vi "Receive DS Packet.vi"(0 "Recv Socket":refnum<k16>, 5 "Log User Data":bool) -> (2 "New Dashboard Data":bool, 3 "Battery":sgl, 4 "Error Strings":string, 6 "Driver Station":T1, 8 "Robot IP Address":string="10.0.0.2", 10 "Status":T3, 12 "Camera IP Address":string="10.0.0.2", 13 "Low Priority User Data":string, 14 "High Priority User Data":string, 15 "Error":T2)   [LabVIEW 2014]
uses:
  DStoPCPacketTypeDef.ctl
panel:
  out "CRC":string
  out "Team ID":u16
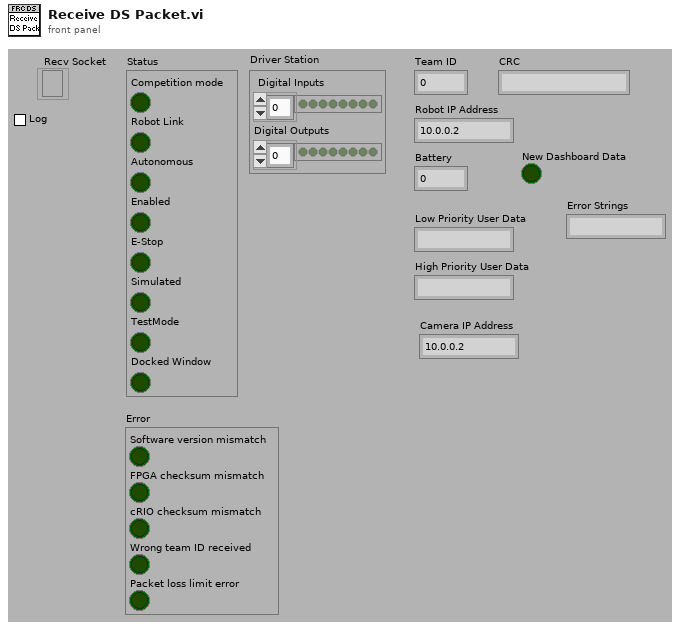
[diagram p1: front panel]
types:
  T1 = cluster{"Digital Inputs":bool[], "Digital Outputs":bool[]}
  T2 = cluster{"Software version mismatch":bool, "FPGA checksum mismatch":bool, "cRIO checksum mismatch":bool, "Wrong team ID received":bool, "Packet loss limit error":bool}
  T3 = cluster{"Competition mode":bool, "Robot Link":bool, "Autonomous":bool, "Enabled":bool, "E-Stop":bool, "Simulated":bool, "TestMode":bool, "Docked Window":bool}
  T4 = typedef "DStoPCPacketTypeDef.ctl" = cluster{"Packet Index":u16, "Digital Inputs":u8, "Digital Out":u8, "Battery":u16, "Status":u8, "Error":u8, "Team ID":u16, "VersionMonth1":u8, "VersionMonth2":u8, "VersionDay1":u8, "VersionDay2":u8, "VersionYear1":u8, "VersionYear2":u8, "Revision1":u8, "Revision2":u8, "Robot IP":u32, "UnusedBuffer 2":u8, "ExtraModeFlags":u8, "Reply Packet #":u16}
  T5 = cluster{"Boolean array":bool[], "Boolean array":bool[]}
  T6 = cluster{"Boolean array[0]":bool, "Boolean array[1]":bool, "Boolean array[2]":bool, "Boolean array[3]":bool, "Boolean array[4]":bool, "Boolean array[5]":bool, "Boolean array[6]":bool, "Boolean array[7]":bool}
  T7 = cluster{"Boolean array[0]":bool, "Boolean array[1]":bool, "Boolean array[4]":bool, "Boolean array[5]":bool, bool, bool, bool, bool}
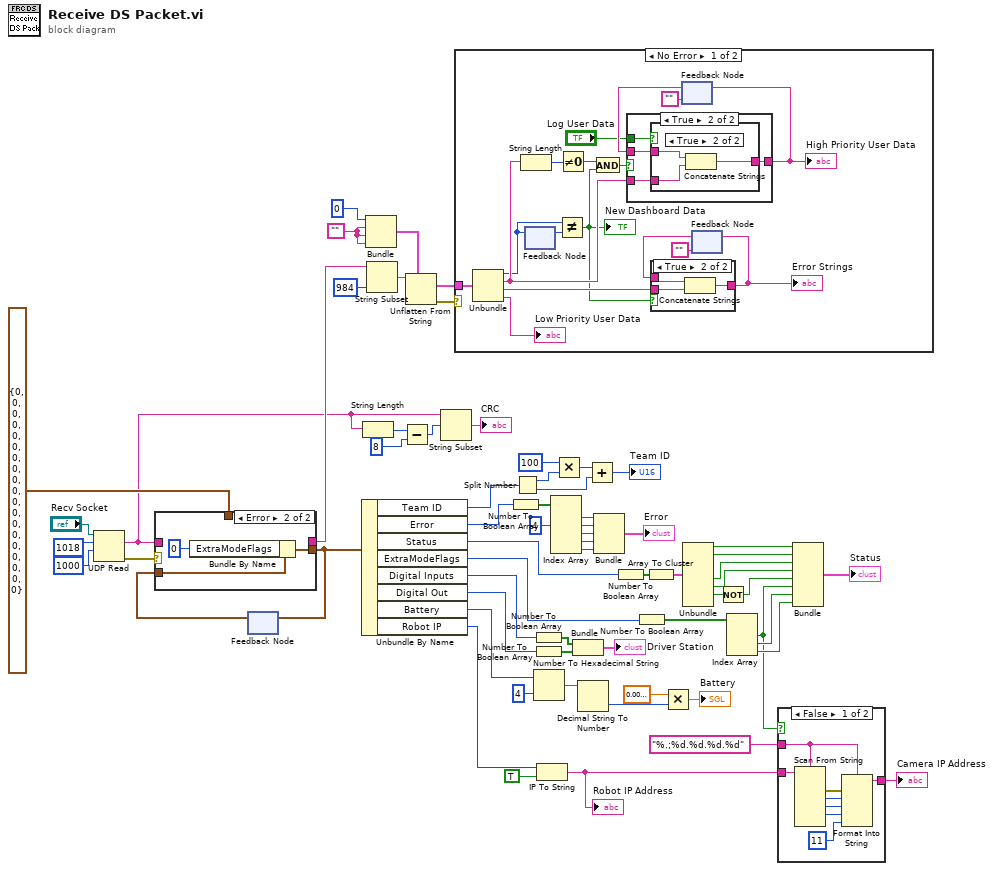
[diagram p0: block diagram]
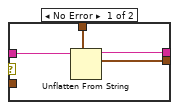
[diagram p2: hidden frame]
diagram:
  w16 = ""
  n1 = UDP Read(connection ID="Recv Socket", max size (548)=1018 ("bytes to read"), timeout ms (25000)=1000) -> (data out=w2:string, error out=w6:errorcluster)  [unwired: 1 in, 3 out]
  n2 = feedback #1() -> (w5:T4)  [unwired: 1 in]
  n3 = case shown="Error" w6 {
    tunnel: w2 -> [w70 _]
    tunnel: w5 -> [_ w72]
    tunnel: [w69 w73] -> w1
    tunnel: T4 {"Packet Index"=0, "Digital Inputs"=0, "Digital Out"=0, "Battery"=0, "Status"=0, "Error"=0, "Team ID"=0, "VersionMonth1"=0, "VersionMonth2"=0, "VersionDay1"=0, "VersionDay2"=0, "VersionYear1"=0, "VersionYear2"=0, "Revision1"=0, "Revision2"=0, "Robot IP"=0, "UnusedBuffer 2"=0, "ExtraModeFlags"=0, "Reply Packet #"=0} ("Cluster") -> [w68 _]
    tunnel: [w67 _] -> w3
    frame No Error {
      n4 = Unflatten From String(type=w68, binary string=w70) -> (rest of the binary string=w67:string, value=w69:T4)  [unwired: 1 in, 3 out]
    }
    frame Error {
      n5 = Bundle By Name(cluster=w72, "ExtraModeFlags"=u8 0) -> (w73:T4)
    }
  }
  n6 = feedback-in #1(w1) -> ()
  n7 = Unbundle By Name(w1) -> ("Team ID"=w50:u16, "Error"=w58:u8, "Status"=w66:u8, "ExtraModeFlags"=w15:u8, "Digital Inputs"=w24:u8, "Digital Out"=w23:u8, "Battery"=w42:u16, "Robot IP"=w7:u32)
  n8 = String Length(string=w2) -> (length=w47:i32)
  n9 = Bundle(u8 0, w16, w16, w16) -> (w20:cluster{u8, string, string, string})  [unwired: 1 out]
  n10 = String Subset(string=w3, length (rest)=984 ("length (rest)")) -> (substring=w25:string)  [unwired: 1 out]
  n11 = Subtract(x=w47, y=8) -> (x-y=w45:i32)
  n12 = Unflatten From String(type=w20, binary string=w25) -> (value=w18:cluster{u8, string, string, string}, error out=w17:errorcluster)  [unwired: 1 in, 3 out]
  n13 = String Subset(string=w2, offset (0)=w45) -> (substring=→"CRC":string)  [unwired: 1 out]
  n14 = case shown="No Error" w17 {
    tunnel: w18 -> [w87 _]
    frame No Error {
      n15 = Unbundle(w87) -> (w78:u8, w79:string, w85:string, →"Low Priority User Data":string)
      n16 = String Length(string=w79) -> (length=w80:i32)
      n17 = feedback-in #2(w78) -> ()
      n18 = feedback #2() -> (w77:u8)  [unwired: 1 out]
      n19 = Not Equal?(x=w78, y=w77) -> (x != y?=w76:bool)
      "New Dashboard Data" <- w76
      n20 = Not Equal To 0?(x=w80) -> (x != 0?=w81:bool)
      n21 = And(x=w81, y=w76) -> (x .and. y?=w82:bool)
      n22 = feedback #3("") -> (w88:string)
      n23 = case shown="True" w82 {
        tunnel: w79 -> [_ w99]
        tunnel: [w95 w98] -> w74
        tunnel: w88 -> [w95 w97]
        tunnel: "Log User Data" -> [_ w96]
        frame False {
        }
        frame True {
          n24 = case shown="True" w96 {
            tunnel: w99 -> [w100 w103]
            tunnel: [w100 w102] -> w98
            tunnel: w97 -> [_ w101]
            frame False {
            }
            frame True {
              n25 = Concatenate Strings(w101, w103) -> (w102:string)
            }
          }
        }
      }
      "High Priority User Data" <- w74
      n26 = feedback-in #3(w74) -> ()
      n27 = feedback #4("") -> (w90:string)
      n28 = case shown="True" w76 {
        tunnel: [w91 w94] -> w75
        tunnel: w90 -> [w91 w93]
        tunnel: w85 -> [_ w92]
        frame False {
        }
        frame True {
          n29 = Concatenate Strings(w93, w92) -> (w94:string)
        }
      }
      "Error Strings" <- w75
      n30 = feedback-in #4(w75) -> ()
    }
    frame Error {
    }
  }
  n31 = Number To Boolean Array(number=w58) -> (Boolean array=w32:bool[])
  n32 = Split Number(x=w50) -> (hi(x)=w55:u8, lo(x)=w52:u8)
  n33 = Number To Boolean Array(number=w24) -> (Boolean array=w21:bool[])
  n34 = Number To Boolean Array(number=w23) -> (Boolean array=w22:bool[])
  n35 = Number To Hexadecimal String(1:i16 4 ("width (-)"), 2:w42) -> (0:w41:string)
  n36 = IP To String(1:TRUE ("dot notation? (F)"), 2:w7) -> (0:w9:string)
  "Robot IP Address" <- w9
  n37 = Index Array(array=w32, index #2=4 ("index")) -> (element #1=w26:bool, element #2=w27:bool, element #3=w28:bool, element #4=w29:bool, element #5=w30:bool)  [unwired: 4 in]
  n38 = Multiply(x=u16 100, y=w55) -> (x*y=w53:u16)
  n39 = Bundle("Boolean array"=w21, "Boolean array"=w22) -> (→"Driver Station":T5)  [unwired: 1 out]
  n40 = Decimal String To Number(string=w41) -> (number=w39:i32)  [unwired: 3 out]
  n41 = Add(x=w53, y=w52) -> (x+y=→"Team ID":u16)
  n42 = Bundle(w26, w27, w28, w29, w30) -> (→"Error":cluster{bool, bool, bool, bool, bool})  [unwired: 1 out]
  n43 = Number To Boolean Array(number=w66) -> (Boolean array=w65:bool[])
  n44 = Number To Boolean Array(number=w15) -> (Boolean array=w14:bool[])
  n45 = Array To Cluster(array=w65) -> (cluster=w63:T6)
  n46 = Multiply(x=sgl 0.01, y=w39) -> (x*y=→"Battery":sgl)
  n47 = Unbundle(w63) -> ("Boolean array[0]"=w62:bool, "Boolean array[1]"=w61:bool, "Boolean array[4]"=w60:bool, "Boolean array[5]"=w59:bool, "Boolean array[6]"=w57:bool)  [unwired: 3 out]
  n48 = Not(x=w57) -> (.not. x?=w56:bool)
  n49 = Index Array(array=w14) -> (element #1=w10:bool, element #2=w13:bool, element #3=w12:bool)  [unwired: 3 in]
  n50 = case shown="False" w10 {
    tunnel: [w106 w112] -> w11
    tunnel: w9 -> [w105 w112]
    tunnel: "%.;%d.%d.%d.%d" ("format string") -> [w104 _]
    frame False {
      n51 = Scan From String(format string=w104, input string=w105) -> (error out=w108:errorcluster, output 1=w109:i32, output 2=w110:i32, output 3=w111:i32)  [unwired: 2 in, 7 out]
      n52 = Format Into String(format string=w104, error in=w108, w109, w110, w111, 11 ("IP Suffix:")) -> (resulting string=w106:string)  [unwired: 1 in, 1 out]
    }
    frame True {
    }
  }
  "Camera IP Address" <- w11
  n53 = Bundle("Boolean array[0]"=w62, "Boolean array[1]"=w61, "Boolean array[4]"=w60, "Boolean array[5]"=w59, w56, w10, w13, w12) -> (→"Status":T7)  [unwired: 1 out]
